vi "Pop state off string queue 2.vi"(7 "Default state":string="User action?", 8 "error in (no error)":errorcluster, 10 "State que in":string[](array[string])) -> (0 "error out":errorcluster, 1 "Not Exit?":bool, 2 "State que out":string[](array[string]), 3 "State case":string)   [LabVIEW 2010]
doc: "Removes the first element of the state que in array. If error in = T then the state case output is \"error\". If queue is empty the output is the \"defualt state\"."
panel:
  # "Error"
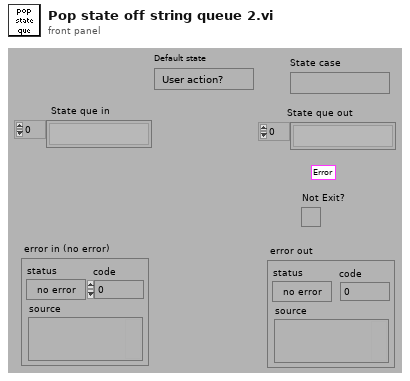
[diagram p1: front panel]
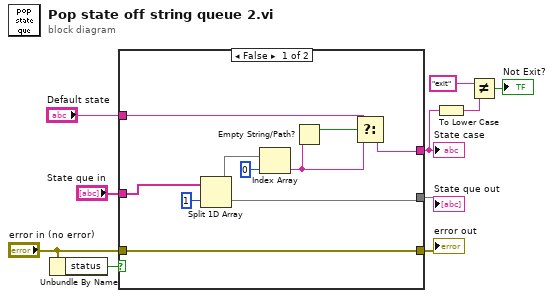
[diagram p0: block diagram]
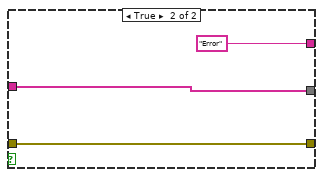
[diagram p2: hidden frame]
diagram:
  n1 = Unbundle By Name("error in (no error)") -> ("status"=w9:bool)
  n2 = case shown="False" w9 {
    tunnel: [w16 w23] -> w8
    tunnel: "error in (no error)" -> [w16 w23]
    tunnel: [w11 "Error"] -> w4
    tunnel: [w20 w22] -> w6
    tunnel: "State que in" -> [w15 w22]
    tunnel: "Default state" -> [w14 _]
    frame False {
      n3 = Split 1D Array(array=w15, index=1) -> (first subarray=w19:string[], second subarray=w20:string[])
      n4 = Index Array(array=w19, index=0) -> (element=w13:string)
      n5 = Empty String/Path?(string/path=w13) -> (empty?=w12:bool)
      n6 = Select(t=w14, s=w12, f=w13) -> (s? t:f=w11:string)
    }
    frame True {
    }
  }
  "error out" <- w8
  "State case" <- w4
  "State que out" <- w6
  n7 = To Lower Case(string=w4) -> (all lower case string=w3:string)
  n8 = Not Equal?(x="exit", y=w3) -> (x != y?=→"Not Exit?":bool)
